vi "Die.vi"() -> ()   [LabVIEW 2011]
panel:
  out "Ring":u16(ring)
  in  "stop":bool
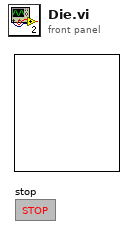
[diagram p1: front panel]
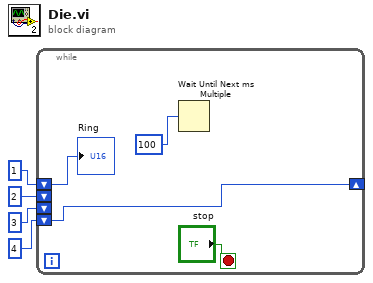
[diagram p0: block diagram]
diagram:
  n1 = while {
    shift-right: [w7] -> _
    shift-left: 1 -> [w5]
    shift-left: 2 -> [_]
    shift-left: 3 -> [_]
    shift-left: 4 -> [w7]
    stop <- "stop" stop-if-true
    n2 = Wait Until Next ms Multiple(millisecond multiple=u32 100) -> ()  [unwired: 1 out]
    "Ring" <- w5
  }
